vi "combiningstring.vi"() -> ()   [LabVIEW 2019]
panel:
  out "concatenated string":string
  in  "String 4":string
  in  "String 3":string
  in  "String 2":string
  in  "String":string
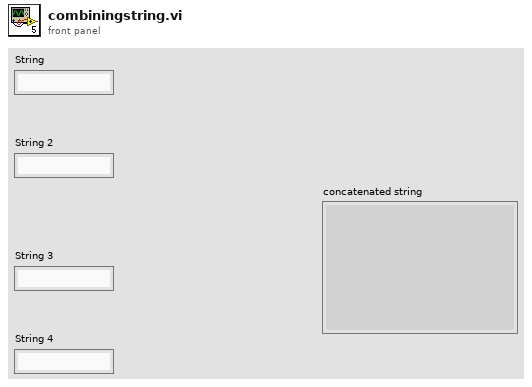
[diagram p1: front panel]
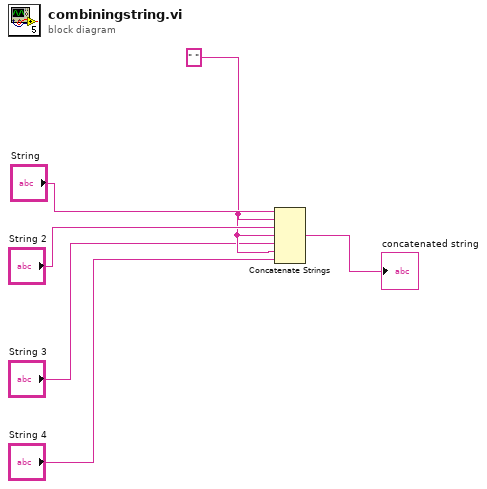
[diagram p0: block diagram]
diagram:
  w4 = " " ("string")
  n1 = Concatenate Strings("String", w4, "String 2", w4, "String 3", w4, "String 4") -> (→"concatenated string":string)
